vi "Get Popout Event.vi"(8 "error in (no error)":errorcluster, 11 "NavPanel in":refnum<class "NavPanel.lvclass">) -> (0 "error out":errorcluster, 2 "Popout Nav Event":refnum<user-event>, 3 "NavPanel out":refnum<class "NavPanel.lvclass">)   [LabVIEW 2020, in "PicoG-App.lvlib" / "NavPanel.lvclass"]
uses:
  NavPanel.lvclass
  <vilib>/IlluminatedG/IG OOPanel/OOPanel/Panel/Panel.lvclass
  Popout Nav Panel Event.ctl
  PicoG-App.lvlib
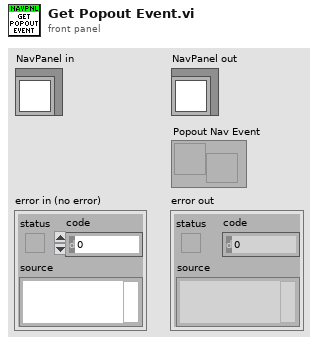
[diagram p1: front panel]
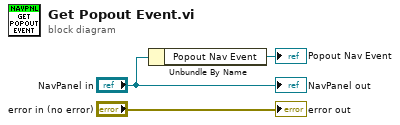
[diagram p0: block diagram]
diagram:
  n1 = Unbundle By Name("NavPanel in") -> ("Popout Nav Event"=→"Popout Nav Event":refnum<user-event>)
  "error out" <- "error in (no error)"
  "NavPanel out" <- "NavPanel in"
